vi "AcquisitionThread.vi"(8 "error in (no error)":errorcluster, 11 "Application Data":T1) -> (0 "error out":errorcluster)   [LabVIEW 2019]
uses:
  Typedefs/#cluster_ApplicationData.ctl
  Typedefs/Acquisition Thread/#cluster_AcqQueueData.ctl
  Typedefs/Acquisition Thread/#enum_AcquisitionTask.ctl
  Typedefs/Saving Thread/#cluster_SavingQueueData.ctl
  Typedefs/Saving Thread/#enum_SavingTask.ctl
  Typedefs/Acquisition Thread/#cluster_AcqThreadData.ctl
  <vilib>/MagicBox/Device/Arduino/Arduino.lvclass
  <vilib>/MagicBox/Peripherals/POX/POX.lvclass
  Typedefs/Acquisition Thread/#enum_AcqThreadState.ctl
  Typedefs/#cluster_GUIRefs.ctl
  LowLevelError.vi
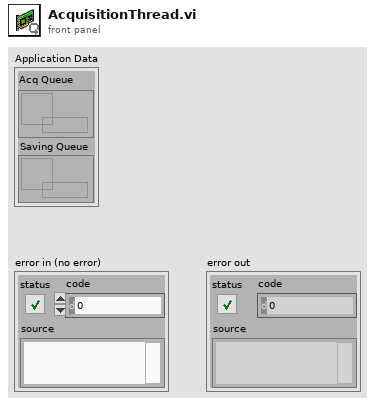
[diagram p1: front panel]
types:
  T1 = typedef "#cluster_ApplicationData.ctl" = cluster{"Acq Queue":refnum<queue>, "Saving Queue":refnum<queue>}
  T2 = typedef "#cluster_AcqThreadData.ctl" = cluster{"Save?":bool, "Arduino":refnum<class "Arduino.lvclass">, "POX":refnum<class "POX.lvclass">, "State":T3, "GUI Refs":T4}
  T3 = typedef "#enum_AcqThreadState.ctl" = enum16{"Idle", "Operate", "Error"}
  T4 = typedef "#cluster_GUIRefs.ctl" = cluster{"Measure":refnum<vi>, "Save?":refnum<vi>, "Stop":refnum<vi>, "Measurement Dir":refnum<vi>, "Heart beat":refnum<vi>, "O2":refnum<vi>, "POX Data History":refnum<vi>}
  T5 = typedef "#cluster_AcqQueueData.ctl" = cluster{"Task":T6, "Data":variant}
  T6 = typedef "#enum_AcquisitionTask.ctl" = enum16{"Init", "Start", "Finish", "Close"}
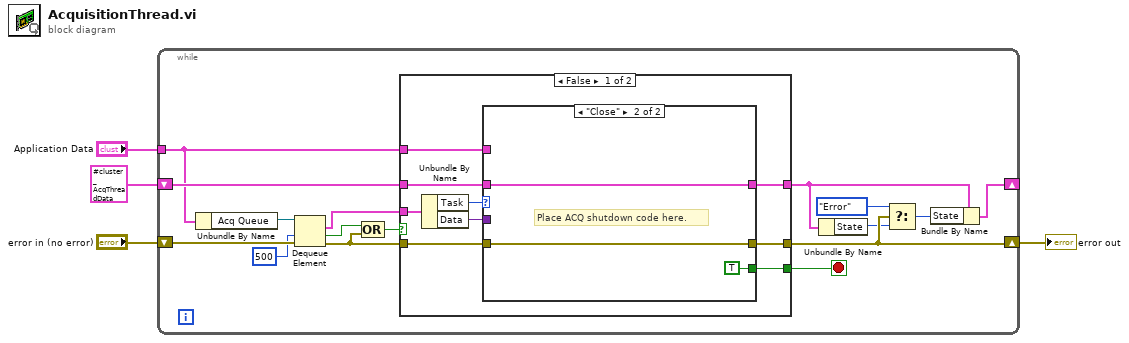
[diagram p0: block diagram]
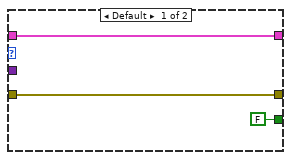
[diagram p2: hidden frame]
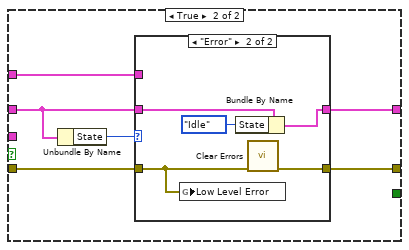
[diagram p3: hidden frame]
diagram:
  n1 = while {
    tunnel: "Application Data" -> [w15]
    shift-right: [w10] -> w2
    shift-left: "error in (no error)" -> [w20]
    shift-right: [w6] -> _
    shift-left: T2 {"Save?"=FALSE, "Arduino"=refnum, "POX"=refnum, "State"=enum."Idle", "GUI Refs"={"Measure"=refnum, "Save?"=refnum, "Stop"=refnum, "Measurement Dir"=refnum, "Heart beat"=refnum, "O2"=refnum, "POX Data History"=refnum}} ("Acq Thread Data") -> [w16]
    stop <- w17 stop-if-true
    n2 = Unbundle By Name(w15) -> ("Acq Queue"=w19:refnum<queue>)
    n3 = Dequeue Element(queue=w19, timeout in ms (-1)=500, error in (no error)=w20) -> (element=w18:T5, timed out?=w13:bool, error out=w11:errorcluster)  [unwired: 1 out]
    n4 = Compound Arithmetic op=OR(w13, w11) -> (w12:bool)
    n5 = case shown="False" w12 {
      tunnel: w18 -> [w29 _]
      tunnel: w11 -> [w26 w41]
      tunnel: [w25 _] -> w17
      tunnel: w16 -> [w24 w39]
      tunnel: [w23 w37] -> w7
      tunnel: w15 -> [w22 w38]
      tunnel: [w21 w36] -> w10
      frame False {
        n6 = Unbundle By Name(w29) -> ("Task"=w28:T6, "Data"=w27:variant)
        n7 = case shown="\"Close\"" w28 {
          tunnel: w27 -> [_ _]
          tunnel: w26 -> [w32 w34]
          tunnel: [w31 w33] -> w23
          tunnel: [FALSE TRUE] -> w25
          tunnel: w24 -> [w31 w33]
          tunnel: w22 -> [_ _]
          tunnel: [w32 w34] -> w21
          frame Default {
          }
          frame "Close" {
            # "Place ACQ shutdown code here."
          }
        }
      }
      frame True {
        n8 = Unbundle By Name(w39) -> ("State"=w40:T3)
        n9 = case shown="\"Error\"" w40 {
          tunnel: w41 -> [w42 w44]
          tunnel: w39 -> [w43 w48]
          tunnel: [w42 w45] -> w36
          tunnel: w38 -> [_ _]
          tunnel: [w43 w47] -> w37
          frame Default {
          }
          frame "Error" {
            n10 = global write "LowLevelError.vi" "Low Level Error"(w44) -> ()
            n11 = Bundle By Name(cluster=w48, "State"=#enum_AcqThreadState."Idle") -> (w47:T2)
            n12 = call <vilib>:"Clear Errors.vi"("error in (no error)"=w44) -> ("error out"=w45:errorcluster)  [unwired: 5 in, 1 out]
          }
        }
      }
    }
    n13 = Unbundle By Name(w7) -> ("State"=w9:T3)
    n14 = Select(t=#enum_AcqThreadState."Error", s=w10, f=w9) -> (s? t:f=w5:T3)
    n15 = Bundle By Name(cluster=w7, "State"=w5) -> (w6:T2)
  }
  "error out" <- w2
